vi "calculatex.vi"(9 "T":dbl, 10 "T0":dbl) -> (2 "X":dbl)   [LabVIEW 2012]
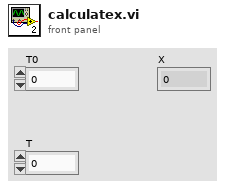
[diagram p1: front panel]
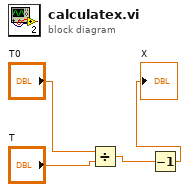
[diagram p0: block diagram]
diagram:
  n1 = Divide(x="T0", y="T") -> (x/y=w2:dbl)
  n2 = Decrement(x=w2) -> (x-1=→"X":dbl)
